vi "Export dat - cDLTS.vi"(8 "Error In":errorcluster, 9 "Workspace":path, 11 "cDLTS measurement":T1={"Name"="", "Comment"="", "Time"=timestamp(0 s since 1904-01-01), "Folder"=path "", "DLTS properties"={"Tstart"=100.0, "Instant start"=FALSE, "Tstop"=350.0, "T rate"=0.016666666666666666, "Test signal"=0.1, "Test frequency"=100000.0, "Bandwidth"=0.0, "Averaging"=5.0, "Vbias"=-5.0, "Vpulse"=-1.0, "pulse length"=0.1, "Pulse 2"=FALSE, "Vpulse 2"=0.0, "pulse length 2"=0.0, "I range"=-2.0, "V range"=10.0, "Emission rate"=[10.0], "Sampling rate"=107000.0, "Acq. delay"=0.0}, "GUID"=""} {"DLTS properties"."V range" items=["10mV"=0.01, "100mV"=0.1, "1V"=1.0, "10V"=10.0]; "DLTS properties"."I range" items=["10mV"=0.01, "100mV"=0.1, "1V"=1.0, "10V"=10.0]}) -> (0 "Error Out":errorcluster)   [LabVIEW 2019]
doc: "Handles export of a DLTS measurement to a .dat file, displays a GUI window"
uses:
  Type defs/cDLTS measurement Type Def.ctl
  Type defs/DLTS properties Type Def.ctl
  <vilib>/Utility/sysdir.llb/System Directory Type.ctl
  <vilib>/Utility/file.llb/Write Delimited Spreadsheet (string).vi
  <vilib>/Utility/file.llb/Write Delimited Spreadsheet (DBL).vi
panel:
  out "String":string
  in  "Path":path caption="Export file as:"
  in  "Export":bool
  in  "Cancel":bool
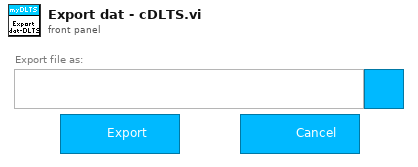
[diagram p1: front panel]
types:
  T1 = typedef "cDLTS measurement Type Def.ctl" = cluster{"Name":string, "Comment":string, "Time":timestamp, "Folder":path, "DLTS properties":T2, "GUID":string}
  T2 = typedef "DLTS properties Type Def.ctl" = cluster{"Tstart":dbl[unit], "Instant start":bool, "Tstop":dbl[unit], "T rate":dbl[unit], "Test signal":dbl[unit], "Test frequency":dbl[unit], "Bandwidth":dbl[unit], "Averaging":dbl, "Vbias":dbl[unit], "Vpulse":dbl[unit], "pulse length":dbl[unit], "Pulse 2":bool, "Vpulse 2":dbl[unit], "pulse length 2":dbl[unit], "I range":dbl, "V range":dbl[unit], "Emission rate":dbl[unit][], "Sampling rate":dbl[unit], "Acq. delay":dbl[unit]}
  T3 = enum32{"existing file", "new file", "new or existing file", "existing dir", "new dir", "new or existing dir", "existing file (use LLBs)", "new file (use LLBs)", "new or existing file (use LLBs)", "new or existing file or directory (use LLBs)", "existing dir (use LLBs)", "new dir (use LLBs)", "new or existing dir (use LLBs)", "existing file or dir", "new file or dir", "new or existing file or dir", "existing file or dir (use LLBs)", "new file or dir (use LLBs)"}
  T4 = typedef "System Directory Type.ctl" = i32
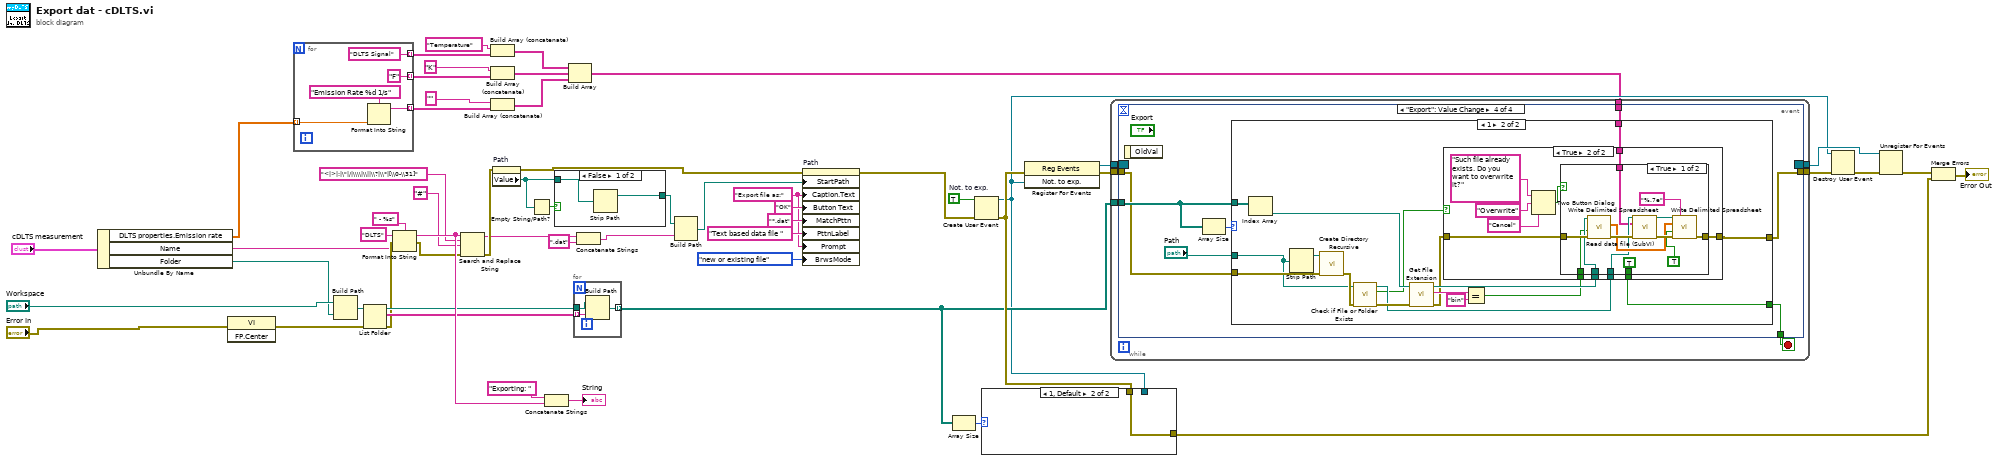
[diagram p0: block diagram]
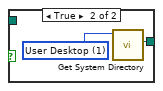
[diagram p2: hidden frame]
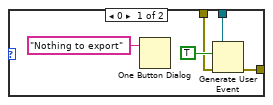
[diagram p3: hidden frame]
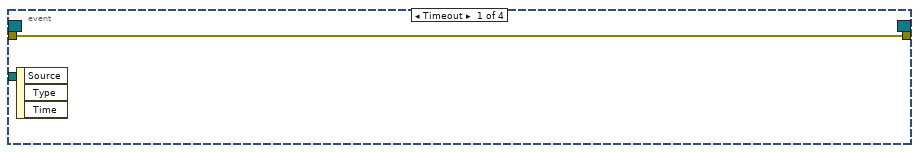
[diagram p4: hidden frame]
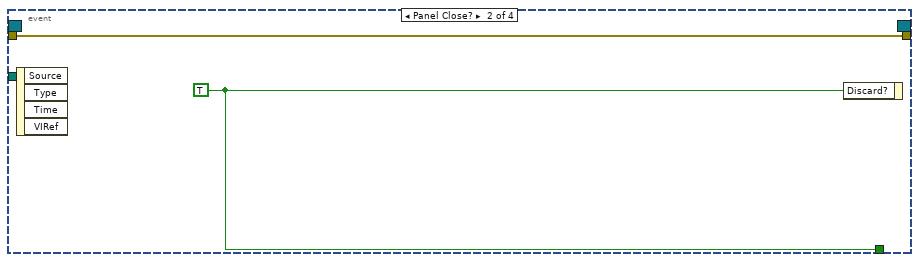
[diagram p5: hidden frame]
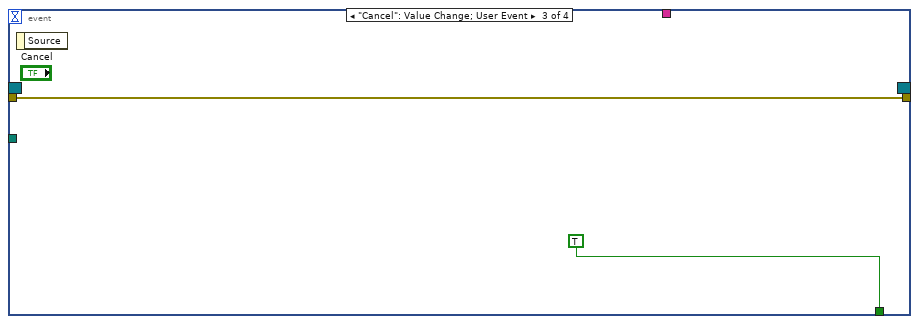
[diagram p6: hidden frame]
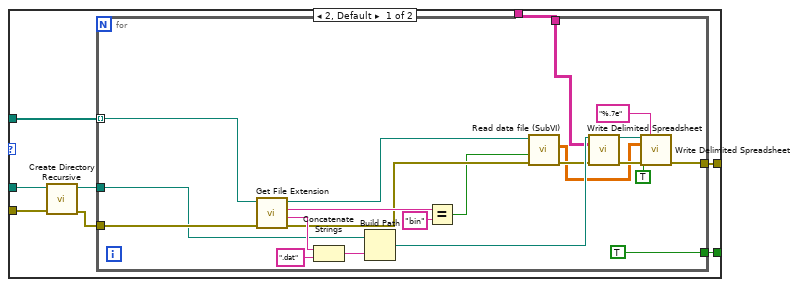
[diagram p7: hidden frame]
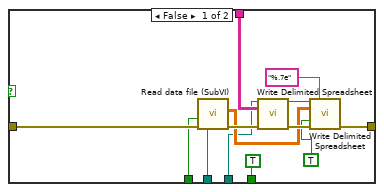
[diagram p8: hidden frame]
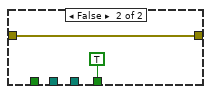
[diagram p9: hidden frame]
diagram:
  w26 = "Export file as:"
  w55 = TRUE  # Not. to exp.
  n1 = Unbundle By Name("cDLTS measurement") -> ("DLTS properties.Emission rate"=w11:dbl[unit][], "Name"=w17:string, "Folder"=w31:path)
  n2 = invoke class="VI" method="FP.Center"(error in="Error In") -> (error out=w13:errorcluster)  [unwired: 2 in, 2 out]
  n3 = for {
    tunnel: w11 -> [w62] mode=indexing
    tunnel: [w60] -> w7 mode=indexing
    tunnel: ["DLTS Signal"] -> w5 mode=indexing
    tunnel: ["F"] -> w6 mode=indexing
    n4 = Format Into String(format string="Emission Rate %d 1/s", w62) -> (resulting string=w60:string)  [unwired: 2 in, 1 out]
  }
  n5 = Build Path(base path="Workspace", name or relative path=w31) -> (appended path=w24:path)
  n6 = List Folder(path=w24, error in=w13) -> (path out=w23:path, filenames=w30:string[], error out=w19:errorcluster)  [unwired: 2 in, 1 out]
  n7 = Format Into String(format string=" - %s", initial string="DLTS", error in=w19, w17) -> (resulting string=w42:string, error out=w18:errorcluster)
  n8 = Search and Replace String(input string=w42, search string="<|>|:|\"|/|\\\\|\\||\\?|\\*|[\\0-\\31]", replace string="#" ("replace string (\"\")"), error in=w18) -> (result string=w16:string, error out=w20:errorcluster)  [unwired: 4 in, 2 out]
  n9 = Build Array (concatenate)("Temperature", w5) -> (w2:string[])
  n10 = Build Array (concatenate)("K", w6) -> (w3:string[])
  n11 = Build Array (concatenate)("", w7) -> (w4:string[])
  n12 = property on="Path" class="Path"(error in=w20) -> (error out=w32:errorcluster, "Value"=w38:path)  [unwired: 1 in, 1 out]
  n13 = Empty String/Path?(string/path=w38) -> (empty?=w39:bool)
  n14 = Concatenate Strings("Exporting: " ("string"), w42) -> (→"String":string)
  n15 = case shown="False" w39 {
    tunnel: w38 -> [w64 _]
    tunnel: [w63 w65] -> w34
    frame False {
      n16 = Strip Path(path=w64) -> (stripped path=w63:path)  [unwired: 1 out]
    }
    frame True {
      w66 = T4 1 items=["User Home"=0, "User Desktop"=1, "User Documents"=2, "User Application Data"=3, "User Preferences"=4, "User Temporary"=5, "Public Documents"=6, "Public Application Data"=7, "Public Preferences"=8, "Public Cache"=13, "System Core Libraries"=9, "System Installed Libraries"=10, "Application Files"=11, "Boot Volume Root"=12] ("system directory type")
      n17 = call <vilib>:"Get System Directory.vi"("system directory type"=w66) -> ("system directory"=w65:path)  [unwired: 10 in]
    }
  }
  n18 = Build Array(w2, w3, w4) -> (w1:string[][])
  n19 = for {
    tunnel: w23 -> [w69]
    tunnel: [w68] -> w50 mode=indexing
    tunnel: w30 -> [w67] mode=indexing
    n20 = Build Path(base path=w69, name or relative path=w67) -> (appended path=w68:path)
  }
  n21 = Concatenate Strings(w16, ".dat" ("string")) -> (w21:string)
  n22 = Build Path(base path=w34, name or relative path=w21) -> (appended path=w33:path)
  n23 = property on="Path" class="Path"(error in=w32, "StartPath"=w33, "Caption.Text"=w26, "Button Text"="OK", "MatchPttn"="*.dat", "PttnLabel"="Text based data file ", "Prompt"=w26, "BrwsMode"=T3."new or existing file" ("Browse Options:Selection Mode")) -> (error out=w52:errorcluster)  [unwired: 1 in, 1 out]
  n24 = Array Size(array=w50) -> (size(s)=w56:i32)
  n25 = Create User Event(user event datatype=w55, error in=w52) -> (user event=w46:refnum<user-event>, error out=w51:errorcluster)
  n26 = case shown="1, Default" w56 {
    tunnel: w46 -> [w73 _]
    tunnel: w51 -> [w71 w75]
    tunnel: [w70 w75] -> w43
    frame 0 {
      n27 = One Button Dialog(message="Nothing to export") -> ()  [unwired: 1 in, 1 out]
      n28 = Generate User Event(user event=w73, event data cluster=TRUE ("event data"), error in=w71) -> (error out=w70:errorcluster)  [unwired: 1 in, 1 out]
    }
    frame 1, Default {
    }
  }
  n29 = register-events(error in=w51, w46) -> (reference out=w53:refnum<event-registration>, error out=w54:errorcluster)  [unwired: 1 in]
  n30 = while {
    tunnel: w54 -> [w82]
    tunnel: [w81] -> w49
    tunnel: w50 -> [w79]
    tunnel: w53 -> [w78]
    tunnel: [w77] -> w47
    tunnel: w1 -> [w76]
    stop <- w80 stop-if-true
    n31 = event shown="[3] \"Export\": Value Change" {
      selector: w78 -> [_ _ _ _]
      dyn-events: [_ _ _ _] -> w77
      timeout: _ -> [_ _ _ _]
      tunnel: w82 -> [w83 w84 w86 w89]
      tunnel: [w83 w84 w86 w94] -> w81
      tunnel: [_ w85 TRUE ("Discard?") w88] -> w80
      tunnel: w79 -> [_ _ _ w92]
      tunnel: w76 -> [_ _ _ w93]
      event Timeout {
        n32 = event-data() -> ()  [unwired: 1 in, 3 out]
      }
      event Panel Close? {
        w85 = TRUE ("Discard?")
        n33 = event-data() -> ()  [unwired: 1 in, 4 out]
        n34 = event-data("Discard?"=w85) -> ()  [unwired: 1 in, 1 out]
      }
      event "Cancel": Value Change; User Event {
        n35 = event-data() -> ()  [unwired: 1 in, 1 out]
      }
      event "Export": Value Change {
        n36 = event-data() -> ()  [unwired: 1 in, 1 out]
        n37 = Array Size(array=w92) -> (size(s)=w91:i32)
        n38 = case shown="1" w91 {
          tunnel: [w102 w131] -> w88
          tunnel: w89 -> [w99 w135]
          tunnel: w92 -> [w101 w134]
          tunnel: "Path" -> [w98 w132]
          tunnel: [w100 w124] -> w94
          tunnel: w93 -> [w95 w125]
          frame 2, Default {
            n39 = call <vilib>:"Create Directory Recursive.vi"("error in (no error)"=w99, "directory"=w98) -> ("error out"=w97:errorcluster, "directory copy"=w96:path)  [unwired: 3 in, 1 out]
            n40 = for {
              tunnel: [TRUE] -> w102
              tunnel: w101 -> [w120] mode=indexing
              tunnel: [w106] -> w100
              tunnel: w97 -> [w116]
              tunnel: w96 -> [w115]
              tunnel: w95 -> [w103]
              n41 = call <vilib>:"Get File Extension.vi"("error in (no error)"=w116, "file"=w120) -> ("error out"=w110:errorcluster, "filename without extension"=w118:string, "lowercase file extension"=w123:string, "dup file"=w111:path)  [unwired: 5 in, 1 out]
              n42 = Concatenate Strings(w118, ".dat" ("string")) -> (w119:string)
              n43 = Build Path(base path=w115, name or relative path=w119) -> (appended path=w108:path)
              n44 = Equal?(x=w123, y="bin") -> (x = y?=w109:bool)
              n45 = call "Read data file (SubVI).vi"("error in"=w110, "Binary"=w109, "file path in"=w111) -> ("error out"=w105:errorcluster, "2D data"=w104:dbl[][])  [unwired: 6 in, 1 out]
              n46 = call-poly <vilib>:"Write Delimited Spreadsheet.vi"("file path (dialog if empty)"=w108, "2D data"=w103, "error in (no error)"=w105) -> ("new file path (Not A Path if cancelled)"=w107:path, "error out"=w113:errorcluster)  [unwired: 11 in]
              n47 = call-poly <vilib>:"Write Delimited Spreadsheet.vi"("file path (dialog if empty)"=w107, "format (%.3f)"="%.7e", "2D data"=w104, "append to file? (new file:F)"=TRUE, "error in (no error)"=w113) -> ("error out"=w106:errorcluster)  [unwired: 9 in, 1 out]
            }
          }
          frame 1 {
            n48 = Index Array(array=w134) -> (element=w133:path)  [unwired: 1 in]
            n49 = Strip Path(path=w132) -> (stripped path=w137:path)  [unwired: 1 out]
            n50 = call <vilib>:"Create Directory Recursive.vi"("error in (no error)"=w135, "directory"=w137) -> ("error out"=w136:errorcluster)  [unwired: 3 in, 2 out]
            n51 = call <vilib>:"Check if File or Folder Exists.vi"("error in (no error)"=w136, "path"=w132) -> ("error out"=w138:errorcluster, "file or folder exists?"=w127:bool, "dup path"=w130:path)  [unwired: 7 in]
            n52 = call <vilib>:"Get File Extension.vi"("error in (no error)"=w138, "file"=w133) -> ("error out"=w126:errorcluster, "lowercase file extension"=w140:string, "dup file"=w129:path)  [unwired: 5 in, 2 out]
            n53 = Equal?(x=w140, y="bin") -> (x = y?=w128:bool)
            n54 = case shown="True" w127 {
              tunnel: [w146 w164] -> w124
              tunnel: [TRUE w163] -> w131
              tunnel: w126 -> [w144 w158]
              tunnel: w130 -> [w141 w157]
              tunnel: w129 -> [w142 w156]
              tunnel: w128 -> [w143 w155]
              tunnel: w125 -> [w145 w154]
              frame False {
                n55 = call "Read data file (SubVI).vi"("error in"=w144, "Binary"=w143, "file path in"=w142) -> ("error out"=w149:errorcluster, "2D data"=w148:dbl[][])  [unwired: 6 in, 1 out]
                n56 = call-poly <vilib>:"Write Delimited Spreadsheet.vi"("file path (dialog if empty)"=w141, "2D data"=w145, "error in (no error)"=w149) -> ("new file path (Not A Path if cancelled)"=w150:path, "error out"=w152:errorcluster)  [unwired: 11 in]
                n57 = call-poly <vilib>:"Write Delimited Spreadsheet.vi"("file path (dialog if empty)"=w150, "format (%.3f)"="%.7e", "2D data"=w148, "append to file? (new file:F)"=TRUE, "error in (no error)"=w152) -> ("error out"=w146:errorcluster)  [unwired: 9 in, 1 out]
              }
              frame True {
                n58 = Two Button Dialog(message="Such file already exists. Do you want to overwrite it?", 1:"Cancel" ("F button name (\"Cancel\")"), 2:"Overwrite" ("T button name (\"OK\")")) -> (T button?=w159:bool)
                n59 = case shown="True" w159 {
                  tunnel: [w170 w178] -> w164
                  tunnel: [TRUE TRUE] -> w163
                  tunnel: w158 -> [w171 w178]
                  tunnel: w157 -> [w169 _]
                  tunnel: w156 -> [w168 _]
                  tunnel: w155 -> [w167 _]
                  tunnel: w154 -> [w165 _]
                  frame True {
                    n60 = call "Read data file (SubVI).vi"("error in"=w171, "Binary"=w167, "file path in"=w168) -> ("error out"=w173:errorcluster, "2D data"=w172:dbl[][])  [unwired: 6 in, 1 out]
                    n61 = call-poly <vilib>:"Write Delimited Spreadsheet.vi"("file path (dialog if empty)"=w169, "2D data"=w165, "error in (no error)"=w173) -> ("new file path (Not A Path if cancelled)"=w174:path, "error out"=w176:errorcluster)  [unwired: 11 in]
                    n62 = call-poly <vilib>:"Write Delimited Spreadsheet.vi"("file path (dialog if empty)"=w174, "format (%.3f)"="%.7e", "2D data"=w172, "append to file? (new file:F)"=TRUE, "error in (no error)"=w176) -> ("error out"=w170:errorcluster)  [unwired: 9 in, 1 out]
                  }
                  frame False {
                  }
                }
              }
            }
          }
        }
      }
    }
  }
  n63 = Destroy User Event(user event=w46, error in=w49) -> (error out=w48:errorcluster)
  n64 = Unregister For Events(event registration refnum=w47, error in=w48) -> (error out=w45:errorcluster)
  n65 = Merge Errors(w45, w43) -> (→"Error Out":errorcluster)
